vi "Get suppressed lines.vi"(8 "error in (no error)":errorcluster, 11 "TTL in":refnum<class "TTL.lvclass">) -> (0 "error out":errorcluster, 2 "Suppressed lines":u8[](array[numeric]), 3 "TTL out":refnum<class "TTL.lvclass">)   [LabVIEW 2011, in "TTL.lvclass"]
uses:
  TTL.lvclass
  TTL.lvclass/TTL.ctl
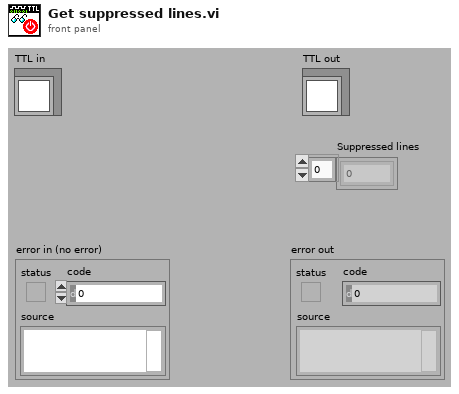
[diagram p1: front panel]
types:
  T1 = typedef "TTL.lvclass/TTL Status Data.ctl" = cluster{"Line states before suppression":bool[], "Suppressed lines":bool[]}
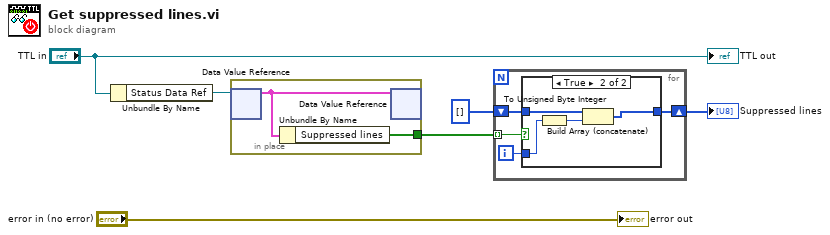
[diagram p0: block diagram]
diagram:
  n1 = Unbundle By Name("TTL in") -> ("Status Data Ref"=w2:refnum<data-value>)
  n2 = in-place {
    in-place-border: [w7] -> w1
    n3 = in-place-dvr #1(w2) -> (w8:T1)  [unwired: 1 out]
    n4 = Unbundle By Name(w8) -> ("Suppressed lines"=w7:bool[])
    n5 = in-place-dvr #1(w8) -> ()  [unwired: 2 out]
  }
  n6 = for {
    tunnel: w1 -> [w12] mode=indexing
    shift-right: [w9] -> w3
    shift-left: u8[] [] -> [w11]
    i -> [w10]
    n7 = case shown="True" w12 {
      tunnel: w11 -> [w13 w17]
      tunnel: w10 -> [_ w15]
      tunnel: [w13 w16] -> w9
      frame False {
      }
      frame True {
        n8 = To Unsigned Byte Integer(number=w15) -> (unsigned 8bit integer=w14:u8)
        n9 = Build Array (concatenate)(w17, w14) -> (w16:u8[])
      }
    }
  }
  "Suppressed lines" <- w3
  "TTL out" <- "TTL in"
  "error out" <- "error in (no error)"
